vi "PPMS.Temperature Status Ring to String.vi"(1 "Temperature Status":T1 items=["TemperatureUnknown"=0, "Stable"=1, "Tracking"=2, "Near"=5, "Chasing"=6, "Filling"=7, "Standby"=10, "Disabled"=13, "ImpedanceNotFunction"=14, "TempFailure"=15]) -> (0 "Status String":string)   [LabVIEW 2019, in "instrument.PPMS.lvclass"]
uses:
  instrument.PPMS.lvclass
  Typedefs/PPMS.Temperature Status--ring.ctl
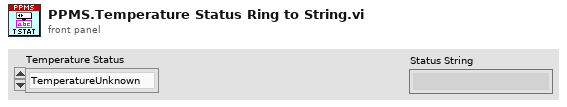
[diagram p1: front panel]
types:
  T1 = typedef "instrument.PPMS.lvclass/PPMS.Temperature Status--ring.ctl" = i32
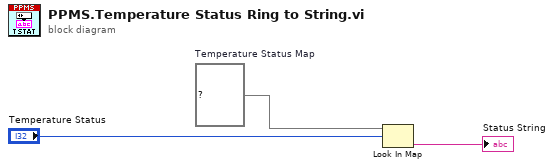
[diagram p0: block diagram]
diagram:
  w1 = map{i32, string} {0="TemperatureUnknown", 1="Stable", 2="Tracking", 5="Near", 6="Chasing", 7="Filling", 10="Standby", 13="Disabled", 14="ImpedanceNotFunction", 15="TempFailure"}  # Temperature Status Map
  n1 = Look In Map(map=w1, key="Temperature Status") -> (value=→"Status String":string)  [unwired: 1 in, 1 out]
